vi "Variant_to_CXT.vi"(8 "Error in":errorcluster, 11 "Value (in)":variant) -> (0 "Error out":errorcluster, 2 "Value (string)":string, 3 "Value (out)":cxt)   [LabVIEW 2012]
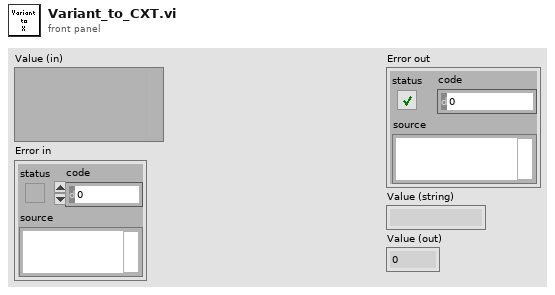
[diagram p1: front panel]
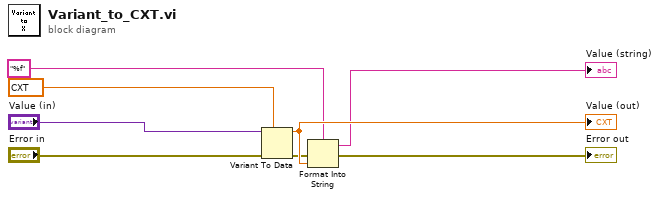
[diagram p0: block diagram]
diagram:
  n1 = Variant To Data(error in="Error in", type=cxt 0.0+0.0i, Variant="Value (in)") -> (data=w7:cxt, error out=w6:errorcluster)
  "Value (out)" <- w7
  n2 = Format Into String(format string="%f", error in=w6, w7) -> (resulting string=→"Value (string)":string, error out=→"Error out":errorcluster)  [unwired: 1 in]
